vi "OP600ZP_DCIR.vi"(3 "tableau":string[][](array[string]), 9 "DCIR_MESURES":T1) -> (2 "Tableau 2":string[][](array[string]), 4 "PASS/FAIL":bool[](array[boolean]))   [LabVIEW 2020]
uses:
  OP600ZP_VGConf.vi
  VG/DCIR@1C.vi
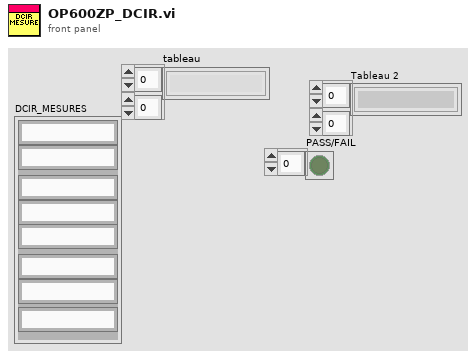
[diagram p1: front panel]
types:
  T1 = cluster{string, string, string, string, string, string, string, string}
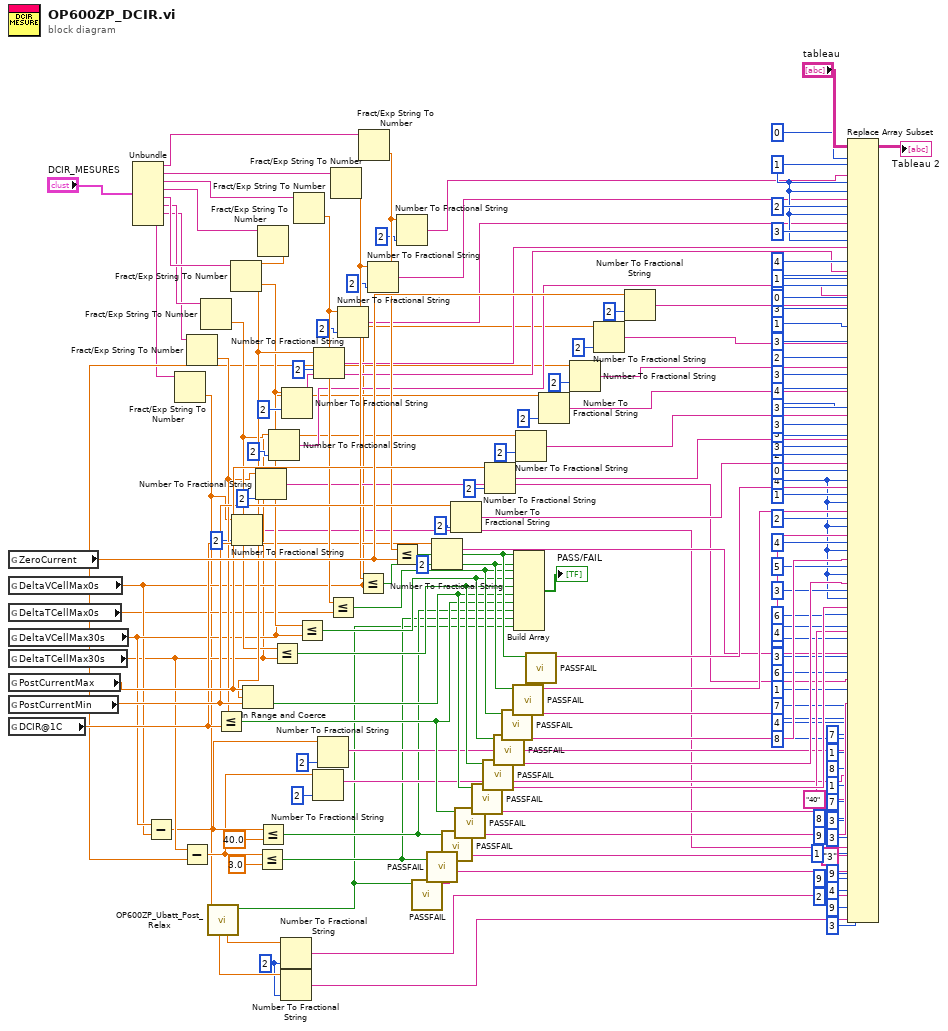
[diagram p0: block diagram]
diagram:
  w7 = i16 2 ("précision (6)")
  w85 = 4 ("indice désactivé (col)")
  w106 = 1 ("indice désactivé (col)")
  n1 = global read "OP600ZP_VGConf.vi" "ZeroCurrent"() -> (w135:dbl)
  n2 = global read "OP600ZP_VGConf.vi" "DeltaVCellMax0s"() -> (w48:dbl)
  n3 = global read "OP600ZP_VGConf.vi" "DeltaTCellMax0s"() -> (w46:dbl)
  n4 = global read "OP600ZP_VGConf.vi" "DeltaVCellMax30s"() -> (w49:dbl)
  n5 = global read "OP600ZP_VGConf.vi" "DeltaTCellMax30s"() -> (w47:dbl)
  n6 = global read "OP600ZP_VGConf.vi" "PostCurrentMax"() -> (w134:dbl)
  n7 = global read "OP600ZP_VGConf.vi" "PostCurrentMin"() -> (w133:dbl)
  n8 = global read "DCIR@1C.vi" "DCIR@1C"() -> (w60:dbl)
  n9 = Unbundle("DCIR_MESURES") -> (w145:string, w144:string, w143:string, w141:string, w70:string, w67:string, w65:string, w19:string)
  n10 = Subtract(x=w49, y=w48) -> (x-y=w36:dbl)
  n11 = Fract/Exp String To Number(string=w19) -> (number=w17:dbl)  [unwired: 3 in, 1 out]
  n12 = Subtract(x=w47, y=w46) -> (x-y=w35:dbl)
  n13 = Fract/Exp String To Number(string=w65) -> (number=w55:dbl)  [unwired: 3 in, 1 out]
  n14 = Fract/Exp String To Number(string=w67) -> (number=w68:dbl)  [unwired: 3 in, 1 out]
  n15 = call "OP600ZP_Ubatt_Post_Relax.vi"("Ubatt Post Relax"=w17) -> ("Dans la gamme ?"=w16:bool, "MIN"=w8:dbl, "MAX"=w9:dbl)  [unwired: 7 in, 1 out]
  n16 = Less Or Equal?(x=w55, y=w60) -> (x <= y?=w64:bool)
  n17 = Fract/Exp String To Number(string=w70) -> (number=w71:dbl)  [unwired: 3 in, 1 out]
  n18 = Number To Fractional String(number=w17, precision (6)=i16 2 ("précision (6)")) -> (F-format string=w13:string)  [unwired: 2 in]
  n19 = Number To Fractional String(number=w55, precision (6)=i16 2 ("précision (6)")) -> (F-format string=w52:string)  [unwired: 2 in]
  n20 = Less Or Equal?(x=w35, y=3.0) -> (x <= y?=w20:bool)
  n21 = Fract/Exp String To Number(string=w141) -> (number=w74:dbl)  [unwired: 3 in, 1 out]
  n22 = In Range and Coerce(upper limit=w134, x=w74, lower limit=w133) -> (In Range?=w98:bool)  [unwired: 1 out]
  n23 = Less Or Equal?(x=w36, y=40.0) -> (x <= y?=w21:bool)
  n24 = Number To Fractional String(number=w68, precision (6)=i16 2 ("précision (6)")) -> (F-format string=w66:string)  [unwired: 2 in]
  n25 = Less Or Equal?(x=w68, y=w47) -> (x <= y?=w99:bool)
  n26 = Number To Fractional String(number=w8, precision (6)=w7) -> (F-format string=w6:string)  [unwired: 2 in]
  n27 = Number To Fractional String(number=w9, precision (6)=w7) -> (F-format string=w5:string)  [unwired: 2 in]
  n28 = Number To Fractional String(number=w71, precision (6)=i16 2 ("précision (6)")) -> (F-format string=w69:string)  [unwired: 2 in]
  n29 = Fract/Exp String To Number(string=w143) -> (number=w78:dbl)  [unwired: 3 in, 1 out]
  n30 = Less Or Equal?(x=w71, y=w49) -> (x <= y?=w100:bool)
  n31 = Number To Fractional String(number=w35, precision (6)=i16 2 ("précision (6)")) -> (F-format string=w31:string)  [unwired: 2 in]
  n32 = Number To Fractional String(number=w74, precision (6)=i16 2 ("précision (6)")) -> (F-format string=w73:string)  [unwired: 2 in]
  n33 = Number To Fractional String(number=w36, precision (6)=i16 2 ("précision (6)")) -> (F-format string=w34:string)  [unwired: 2 in]
  n34 = Less Or Equal?(x=w78, y=w46) -> (x <= y?=w101:bool)
  n35 = Fract/Exp String To Number(string=w144) -> (number=w81:dbl)  [unwired: 3 in, 1 out]
  n36 = Number To Fractional String(number=w78, precision (6)=i16 2 ("précision (6)")) -> (F-format string=w77:string)  [unwired: 2 in]
  n37 = Less Or Equal?(x=w81, y=w48) -> (x <= y?=w102:bool)
  n38 = Fract/Exp String To Number(string=w145) -> (number=w84:dbl)  [unwired: 3 in, 1 out]
  n39 = Number To Fractional String(number=w81, precision (6)=i16 2 ("précision (6)")) -> (F-format string=w80:string)  [unwired: 2 in]
  n40 = Less Or Equal?(x=w84, y=w135) -> (x <= y?=w103:bool)
  n41 = Number To Fractional String(number=w84, precision (6)=i16 2 ("précision (6)")) -> (F-format string=w83:string)  [unwired: 2 in]
  n42 = call <userlib>:"PASSFAIL.vi"("E"=w16) -> ("S"=w12:string)  [unwired: 10 in]
  n43 = call <userlib>:"PASSFAIL.vi"("E"=w20) -> ("S"=w43:string)  [unwired: 10 in]
  n44 = Number To Fractional String(number=w60, precision (6)=i16 2 ("précision (6)")) -> (F-format string=w58:string)  [unwired: 2 in]
  n45 = call <userlib>:"PASSFAIL.vi"("E"=w21) -> ("S"=w44:string)  [unwired: 10 in]
  n46 = Number To Fractional String(number=w133, precision (6)=i16 2 ("précision (6)")) -> (F-format string=w120:string)  [unwired: 2 in]
  n47 = call <userlib>:"PASSFAIL.vi"("E"=w64) -> ("S"=w63:string)  [unwired: 10 in]
  n48 = call <userlib>:"PASSFAIL.vi"("E"=w98) -> ("S"=w87:string)  [unwired: 10 in]
  n49 = call <userlib>:"PASSFAIL.vi"("E"=w99) -> ("S"=w89:string)  [unwired: 10 in]
  n50 = Number To Fractional String(number=w134, precision (6)=i16 2 ("précision (6)")) -> (F-format string=w107:string)  [unwired: 2 in]
  n51 = call <userlib>:"PASSFAIL.vi"("E"=w100) -> ("S"=w91:string)  [unwired: 10 in]
  n52 = call <userlib>:"PASSFAIL.vi"("E"=w101) -> ("S"=w93:string)  [unwired: 10 in]
  n53 = call <userlib>:"PASSFAIL.vi"("E"=w102) -> ("S"=w95:string)  [unwired: 10 in]
  n54 = Build Array(w103, w102, w101, w100, w99, w98, w64, w21, w20, w16) -> (→"PASS/FAIL":bool[])
  n55 = Number To Fractional String(number=w47, precision (6)=i16 2 ("précision (6)")) -> (F-format string=w121:string)  [unwired: 2 in]
  n56 = call <userlib>:"PASSFAIL.vi"("E"=w103) -> ("S"=w97:string)  [unwired: 10 in]
  n57 = Number To Fractional String(number=w49, precision (6)=i16 2 ("précision (6)")) -> (F-format string=w122:string)  [unwired: 2 in]
  n58 = Number To Fractional String(number=w46, precision (6)=i16 2 ("précision (6)")) -> (F-format string=w123:string)  [unwired: 2 in]
  n59 = Number To Fractional String(number=w48, precision (6)=i16 2 ("précision (6)")) -> (F-format string=w124:string)  [unwired: 2 in]
  n60 = Number To Fractional String(number=w135, precision (6)=i16 2 ("précision (6)")) -> (F-format string=w125:string)  [unwired: 2 in]
  n61 = Replace Array Subset(array="tableau", new element #1=w83, index (row) #1=0 ("indice (ligne)"), index (col) #1=w106, new element #2=w80, index (row) #2=w106, index (col) #2=w106, new element #3=w77, index (row) #3=2 ("indice (ligne)"), index (col) #3=w106, new element #4=w73, index (row) #4=3 ("indice (ligne)"), index (col) #4=w106, new element #5=w69, index (row) #5=4 ("indice (ligne)"), index (col) #5=1 ("indice désactivé (col)"), new element #6=w66, index (row) #6=5 ("indice (ligne)"), index (col) #6=1 ("indice désactivé (col)"), new element #7=w125, index (row) #7=0 ("indice (ligne)"), index (col) #7=3 ("indice désactivé (col)"), new element #8=w124, index (row) #8=1 ("indice (ligne)"), index (col) #8=3 ("indice désactivé (col)"), new element #9=w123, index (row) #9=2 ("indice (ligne)"), index (col) #9=3 ("indice désactivé (col)"), new element #10=w122, index (row) #10=4 ("indice (ligne)"), index (col) #10=3 ("indice désactivé (col)"), new element #11=w121, index (row) #11=5 ("indice (ligne)"), index (col) #11=3 ("indice désactivé (col)"), new element #12=w107, index (row) #12=3 ("indice (ligne)"), index (col) #12=3 ("indice désactivé (col)"), new element #13=w120, index (row) #13=3 ("indice (ligne)"), index (col) #13=2 ("indice désactivé (col)"), new element #14=w97, index (row) #14=0 ("indice (ligne)"), index (col) #14=w85, new element #15=w95, index (row) #15=1 ("indice (ligne)"), index (col) #15=w85, new element #16=w93, index (row) #16=2 ("indice (ligne)"), index (col) #16=w85, new element #17=w91, index (row) #17=4 ("indice (ligne)"), index (col) #17=w85, new element #18=w89, index (row) #18=5 ("indice (ligne)"), index (col) #18=w85, new element #19=w87, index (row) #19=3 ("indice (ligne)"), index (col) #19=w85, new element #20=w63, index (row) #20=6 ("indice (ligne)"), index (col) #20=4 ("indice désactivé (col)"), new element #21=w58, index (row) #21=6 ("indice (ligne)"), index (col) #21=3 ("indice désactivé (col)"), new element #22=w52, index (row) #22=6 ("indice (ligne)"), index (col) #22=1 ("indice désactivé (col)"), new element #23=w44, index (row) #23=7 ("indice (ligne)"), index (col) #23=4 ("indice désactivé (col)"), new element #24=w43, index (row) #24=8 ("indice (ligne)"), index (col) #24=4 ("indice désactivé (col)"), new element #25=w34, index (row) #25=7 ("indice (ligne)"), index (col) #25=1 ("indice désactivé (col)"), new element #26=w31, index (row) #26=8 ("indice (ligne)"), index (col) #26=1 ("indice désactivé (col)"), new element #27="40" ("nouvel élément/sous-tableau"), index (row) #27=7 ("indice (ligne)"), index (col) #27=3 ("indice désactivé (col)"), new element #28="3" ("nouvel élément/sous-tableau"), index (row) #28=8 ("indice (ligne)"), index (col) #28=3 ("indice désactivé (col)"), new element #29=w13, index (row) #29=9 ("indice (ligne)"), index (col) #29=1 ("indice désactivé (col)"), new element #30=w12, index (row) #30=9 ("indice (ligne)"), index (col) #30=4 ("indice désactivé (col)"), new element #31=w6, index (row) #31=9 ("indice (ligne)"), index (col) #31=2 ("indice désactivé (col)"), new element #32=w5, index (row) #32=9 ("indice (ligne)"), index (col) #32=3 ("indice désactivé (col)")) -> (→"Tableau 2":string[][])
